vi "Calculate defocus.vi"(8 "error in (no error)":errorcluster, 11 "Cascade in":refnum<class "Cascade.lvclass">) -> (0 "error out":errorcluster, 1 "fine?":bool, 2 "translation out":dbl[unit], 3 "Cascade out":refnum<class "Cascade.lvclass">)   [LabVIEW 2012, in "Cascade.lvclass"]
uses:
  Cascade.lvclass
  dependencies/ImageReg/Registration method.ctl
  Cascade.lvclass/Cascade.ctl
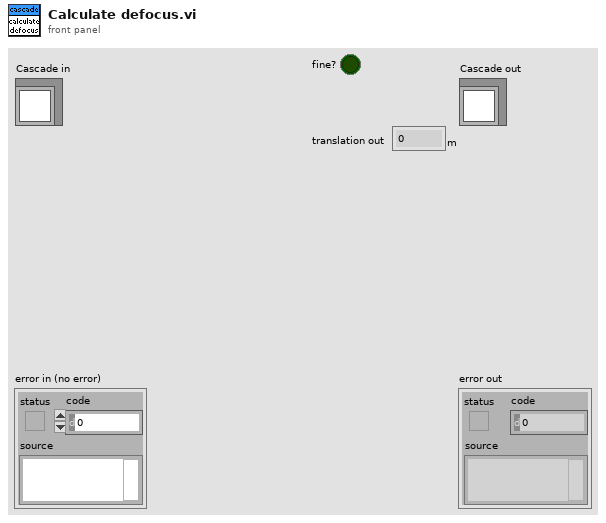
[diagram p1: front panel]
types:
  T1 = typedef "Registration method.ctl" = enum16{"Binarization", "Difference of Gaussians", "Edges Detection", "Gaussians and Binarization", "Edges and Gaussians", "Edges and Binarization", "All"}
  T2 = typedef "IMAQ Image.ctl" = refnum<image>
  T3 = typedef "Gaussian blur parameters.ctl" = cluster{"large sigma":sgl, "small sigma":sgl, "equalize?":bool}
  T4 = typedef "Edge and object parameters.ctl" = cluster{"Canny Edge Parameters":cluster{"Sigma":sgl, "HThresh":sgl, "LThres":sgl, "WindowSize":i32}, "Smoothing parameters":cluster{"X Size":i32, "Y Size":i32, "% Tolerance":i32}, "Dilation iteration":i32, "Object recognition parameters":cluster{"Objects":u16, "Threshold":i32, "Reject Border":bool, "Fill Holes":bool, "Min Object Size":bool, "Min Size":i32, "Max Object Size":bool, "Max Size":i32, "Show Search Area":bool, "Show Center":bool, "Show Bounding Box":bool}}
  T5 = typedef "BinarizationParameters.ctl" = cluster{"threshold percentage":dbl, "equalize?":bool, "Method (clustering)":i32}
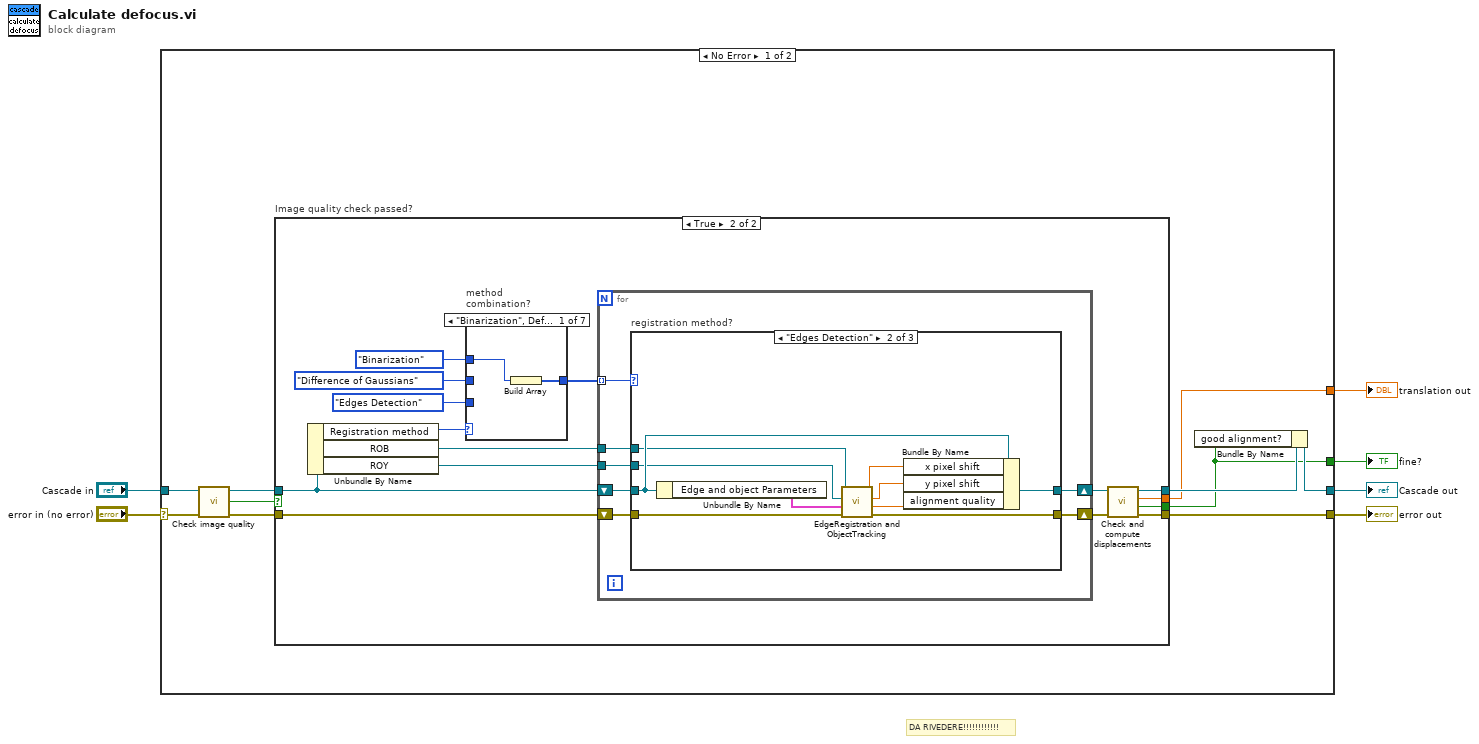
[diagram p0: block diagram]
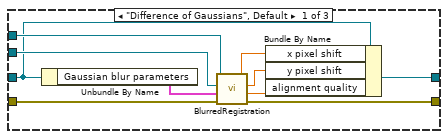
[diagram p3: hidden frame]
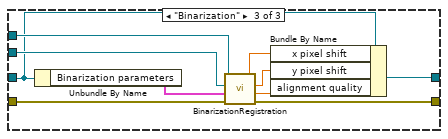
[diagram p4: hidden frame]
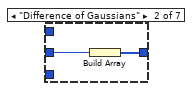
[diagram p5: hidden frame]
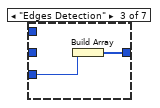
[diagram p6: hidden frame]
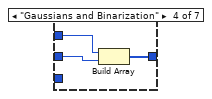
[diagram p7: hidden frame]
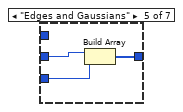
[diagram p8: hidden frame]
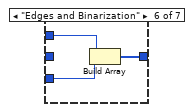
[diagram p9: hidden frame]
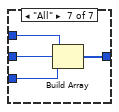
[diagram p10: hidden frame]
diagram:
  # "DA RIVEDERE!!!!!!!!!!!!"
  n1 = case shown="No Error" "error in (no error)" {
    selector: "error in (no error)" -> [w16 w91]
    tunnel: [w11 w91] -> w5
    tunnel: [w10 w90] -> w3
    tunnel: "Cascade in" -> [w15 w90]
    tunnel: [w8 _] -> w2
    tunnel: [w7 _] -> w1
    frame No Error {
      n2 = call-dynamic "Check image quality.vi"("error in (no error)"=w16, "Cascade in"=w15) -> ("error out"=w13:errorcluster, "QC passed?"=w14:bool, "Cascade out"=w12:refnum<class "Cascade.lvclass">)  [unwired: 7 in]
      n3 = case "Image quality check passed?" shown="True" w14 {
        tunnel: w13 -> [w18 w29]
        tunnel: w12 -> [w17 w28]
        tunnel: [w17 w22] -> w9
        tunnel: [w18 w21] -> w11
        tunnel: [_ w20] -> w8
        tunnel: [_ w19] -> w7
        frame False {
        }
        frame True {
          n4 = Unbundle By Name(w28) -> ("Registration method"=w30:T1, "ROB"=w26:T2, "ROY"=w25:T2)
          n5 = case "method\ncombination?" shown="\"Binarization\", Default" w30 {
            tunnel: [w72 w74 w76 w79 w82 w85 w89] -> w27
            tunnel: Registration_method."Difference of Gaussians" ("Registration method") -> [_ w73 _ w77 w81 _ w86]
            tunnel: Registration_method."Binarization" ("Registration method") -> [w71 _ _ w78 _ w83 w88]
            tunnel: Registration_method."Edges Detection" ("Registration method") -> [_ _ w75 _ w80 w84 w87]
            frame "Binarization", Default {
              n6 = Build Array(w71) -> (w72:T1[])
            }
            frame "Difference of Gaussians" {
              n7 = Build Array(w73) -> (w74:T1[])
            }
            frame "Edges Detection" {
              n8 = Build Array(w75) -> (w76:T1[])
            }
            frame "Gaussians and Binarization" {
              n9 = Build Array(w78, w77) -> (w79:T1[])
            }
            frame "Edges and Gaussians" {
              n10 = Build Array(w81, w80) -> (w82:T1[])
            }
            frame "Edges and Binarization" {
              n11 = Build Array(w83, w84) -> (w85:T1[])
            }
            frame "All" {
              n12 = Build Array(w88, w86, w87) -> (w89:T1[])
            }
          }
          n13 = for {
            shift-right: [w37] -> w23
            shift-left: w29 -> [w38]
            shift-right: [w34] -> w24
            shift-left: w28 -> [w39]
            tunnel: w27 -> [w40] mode=indexing
            tunnel: w26 -> [w36]
            tunnel: w25 -> [w35]
            n14 = case "registration method?" shown="\"Edges Detection\"" w40 {
              tunnel: w39 -> [w45 w60 w65]
              tunnel: w38 -> [w50 w58 w70]
              tunnel: [w49 w54 w69] -> w37
              tunnel: w36 -> [w48 w56 w68]
              tunnel: w35 -> [w47 w55 w67]
              tunnel: [w41 w59 w61] -> w34
              frame "Difference of Gaussians", Default {
                n15 = Unbundle By Name(w45) -> ("Gaussian blur parameters"=w46:T3)
                n16 = call "BlurredRegistration.vi"("error in"=w50, "Gaussian blur parameters"=w46, "roy"=w47, "rob"=w48) -> ("error out"=w49:errorcluster, "alignment quality"=w42:dbl, "y displacement"=w43:dbl, "x displacement"=w44:dbl)  [unwired: 4 in]
                n17 = Bundle By Name(cluster=w45, "x pixel shift"=w44, "y pixel shift"=w43, "alignment quality"=w42) -> (w41:refnum<class "Cascade.lvclass">)
              }
              frame "Edges Detection" {
                n18 = Unbundle By Name(w60) -> ("Edge and object Parameters"=w57:T4)
                n19 = call "EdgeRegistration and ObjectTracking.vi"("error in (no error)"=w58, "Edge and object Parameters"=w57, "Roy"=w55, "Rob"=w56) -> ("error out"=w54:errorcluster, "Max value"=w51:dbl, "y translation"=w52:dbl, "x translation"=w53:dbl)  [unwired: 2 in, 2 out]
                n20 = Bundle By Name(cluster=w60, "x pixel shift"=w53, "y pixel shift"=w52, "alignment quality"=w51) -> (w59:refnum<class "Cascade.lvclass">)
              }
              frame "Binarization" {
                n21 = Unbundle By Name(w65) -> ("Binarization parameters"=w66:T5)
                n22 = call "BinarizationRegistration.vi"("error in"=w70, "Binarization parameters"=w66, "Roy"=w67, "Rob"=w68) -> ("error out"=w69:errorcluster, "quality"=w62:dbl, "y translation"=w63:dbl, "x translation"=w64:dbl)  [unwired: 4 in]
                n23 = Bundle By Name(cluster=w65, "x pixel shift"=w64, "y pixel shift"=w63, "alignment quality"=w62) -> (w61:refnum<class "Cascade.lvclass">)
              }
            }
          }
          n24 = call-dynamic "Check and compute displacements.vi"("error in (no error)"=w23, "Cascade in"=w24) -> ("error out"=w21:errorcluster, "fine?"=w20:bool, "translation out"=w19:dbl[unit], "Cascade out"=w22:refnum<class "Cascade.lvclass">)  [unwired: 6 in]
        }
      }
      n25 = Bundle By Name(cluster=w9, "good alignment?"=w8) -> (w10:refnum<class "Cascade.lvclass">)
    }
    frame Error {
    }
  }
  "error out" <- w5
  "Cascade out" <- w3
  "fine?" <- w2
  "translation out" <- w1
